vi "Storage Data.vi"(8 "error in (no error)":errorcluster, 9 "Time Out In ms":i32=-1, 10 "Data in":variant, 11 "2D U16 DVR Array in":refnum<class "2D U16 DVR Array.lvclass">) -> (0 "error out":errorcluster, 1 "Timeout":bool, 3 "2D U16 DVR Array out":refnum<class "2D U16 DVR Array.lvclass">)   [LabVIEW 2024, in "2D U16 DVR Array.lvclass"]
uses:
  2D U16 DVR Array.lvclass
  2D U16 DVR Array.lvclass/2D U16 DVR Array.ctl
  Public Data/Write Count.vi
  Public Data/Read Count.vi
  Public Data/Read Buffer Size.vi
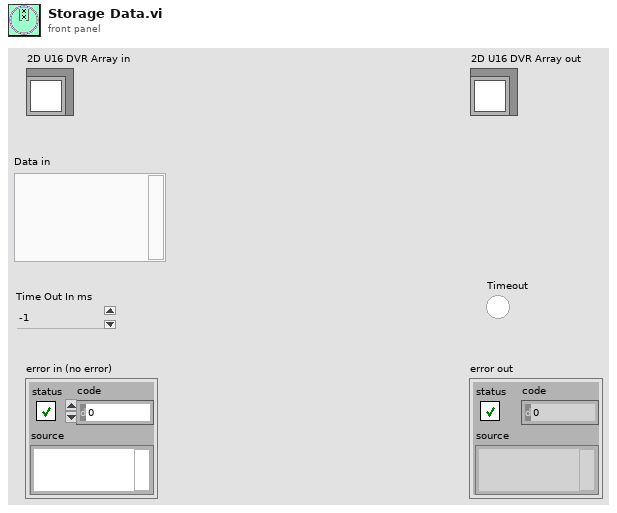
[diagram p1: front panel]
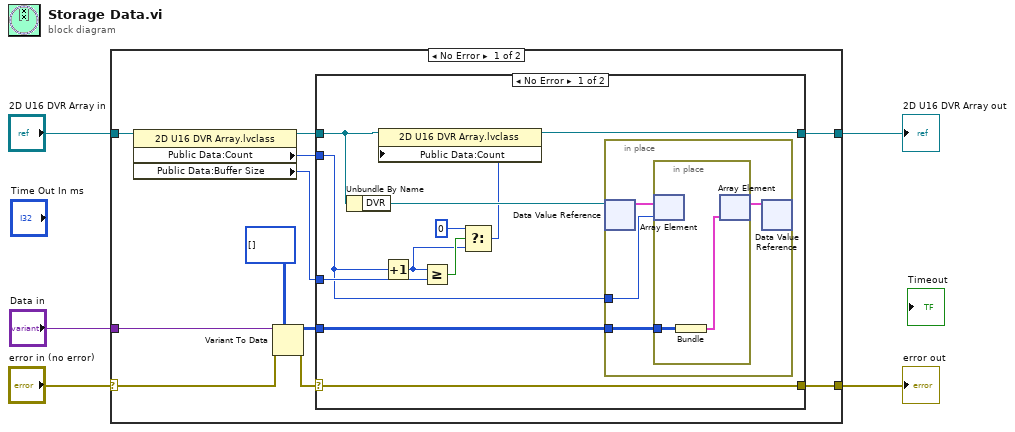
[diagram p0: block diagram]
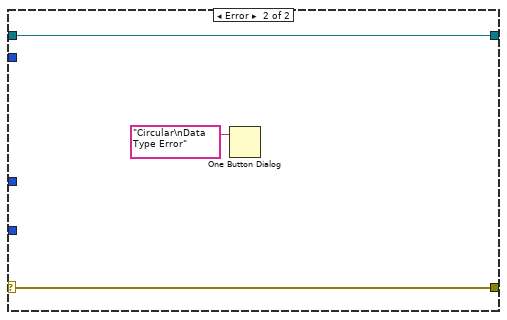
[diagram p2: hidden frame]
diagram:
  n1 = case shown="No Error" "error in (no error)" {
    selector: "error in (no error)" -> [w10 w37]
    tunnel: [w16 w37] -> w5
    tunnel: "2D U16 DVR Array in" -> [w9 w38]
    tunnel: [w15 w38] -> w3
    tunnel: "Data in" -> [w12 _]
    frame No Error {
      n2 = property class="2D U16 DVR Array.lvclass"(reference=w9) -> (reference out=w8:refnum<class "2D U16 DVR Array.lvclass">, "Public Data:Count"=w7:i32, "Public Data:Buffer Size"=w6:i32)  [unwired: 1 in, 1 out]
      n3 = Variant To Data(error in=w10, type=u16[][] [] ("Data In"), Variant=w12) -> (data=w13:u16[][], error out=w11:errorcluster)
      n4 = case shown="No Error" w11 {
        selector: w11 -> [w27 w36]
        tunnel: [w27 w36] -> w16
        tunnel: [w22 w35] -> w15
        tunnel: w8 -> [w23 w35]
        tunnel: w13 -> [w25 _]
        tunnel: w7 -> [w20 _]
        tunnel: w6 -> [w24 _]
        frame No Error {
          n5 = Unbundle By Name(w23) -> ("DVR"=w26:refnum<data-value>)
          n6 = Increment(x=w20) -> (x+1=w19:i32)
          n7 = Greater Or Equal?(x=w19, y=w24) -> (x >= y?=w21:bool)
          n8 = Select(t=0, s=w21, f=w19) -> (s? t:f=w17:i32)
          n9 = property class="2D U16 DVR Array.lvclass"(reference=w23, "Public Data:Count"=w17) -> (reference out=w22:refnum<class "2D U16 DVR Array.lvclass">)  [unwired: 1 in, 1 out]
          n10 = in-place {
            in-place-border: w25 -> [w30]
            in-place-border: w20 -> [w28]
            n11 = in-place-dvr #1(w26) -> (w31:cluster{u16[][]}[])  [unwired: 1 out]
            n12 = in-place {
              in-place-border: w30 -> [w33]
              n13 = in-place-array #2(w31, w28) -> ()  [unwired: 1 out]
              n14 = Bundle("Data In"=w33) -> (w32:cluster{"Data In":u16[][]})  [unwired: 1 in]
              n15 = in-place-array #2(w32) -> (w29:cluster{u16[][]}[])  [unwired: 1 out]
            }
            n16 = in-place-dvr #1(w29) -> ()  [unwired: 2 out]
          }
        }
        frame Error {
          n17 = One Button Dialog(message="Circular\nData Type Error") -> ()  [unwired: 1 in, 1 out]
        }
      }
    }
    frame Error {
    }
  }
  "error out" <- w5
  "2D U16 DVR Array out" <- w3
